vi "Encode_Decode Frame.vi"() -> ()   [LabVIEW 2020]
uses:
  Azdo/emea-aim-664-instrument-driver-1204/src/_controls/queue_data_full.ctl
  Azdo/emea-aim-664-instrument-driver-1204/src/_controls/queue_header_generic.ctl
  <vilib>/addons/_JKI Toolkits/Caraya/classes/Assert/Assert Equal Value_Variant.vi
  Azdo/emea-aim-664-instrument-driver-1204/src/AIM664LV.lvlib
  <vilib>/addons/_JKI Toolkits/Caraya/classes/Test/Test.lvclass
  <vilib>/addons/_JKI Toolkits/Caraya/classes/Assert/Assert.lvclass
panel:
  out "recv size":i32
  out "sent size":i32
  out "sent":u8[](array[numeric])
  out "recvd":u8[](array[numeric])
  in  "HeaderInfo":T1={"InterFrameGap"=0, "PacketGroupWaitTime"=10000, "PayloadBufferMode"=0, "PayloadGenerationMode"=0, "PreambleCount"=7, "Skew"=0, "NetSelect"=4, "FrameStartMode"=1, "PhysErrorInjection"=0, "SequenceNumberInit"=65535, "SequenceNumberOffset"=65535} {"NetSelect" items=["FDX_TX_FRAME_DLY_A"=0, "FDX_TX_FRAME_DLY_B"=1, "FDX_TX_FRAME_BOTH "=3, "FDX_TX_FRAME_ONLY_A"=4, "FDX_TX_FRAME_ONLY_B "=5]; "FrameStartMode" items=["FDX_TX_FRAME_START_IFG", "FDX_TX_FRAME_START_PGWT", "FDX_TX_FRAME_START_TRG"]; "PhysErrorInjection" items=["FDX_TX_FRAME_ERR_OFF"=0, "FDX_TX_FRAME_ERR_CRC"=1, "FDX_TX_FRAME_ERR_ALI"=2, "FDX_TX_FRAME_ERR_PRE"=4, "FDX_TX_FRAME_ERR_PHY"=8]; "SequenceNumberInit" items=["FDX_TX_FRAME_SEQ_INIT_AUTO"=65535]; "SequenceNumberOffset" items=["FDX_TX_FRAME_SEQ_OFFS_AUTO "=65535]; "PayloadGenerationMode" items=["FDX_TX_FRAME_PGM_USER"=0, "FDX_TX_FRAME_PGM_IP_PART"=1, "FDX_TX_FRAME_PGM_IP_FULL"=2, "FDX_TX_FRAME_PGM_IP_PART_TT"=10, "FDX_TX_FRAME_PGM_IP_FULL_TT"=20]; "PayloadBufferMode" items=["FDX_TX_FRAME_PBM_STD", "FDX_TX_FRAME_PBM_MAC", "FDX_TX_FRAME_PBM_UDP"]}
  in  "Frame payload size (bytes)":i32=100
  in  "UDPsrcPort":u16=1
  in  "Frame Configuration":T2={"domainID"=1, "sideID"=1, "locationID"=1, "interfaceID"=1, "partitionID"=1} {"interfaceID" format="%.0b"}
  in  "UDPdstPort":u16=1
  in  "VL Id":u16=60
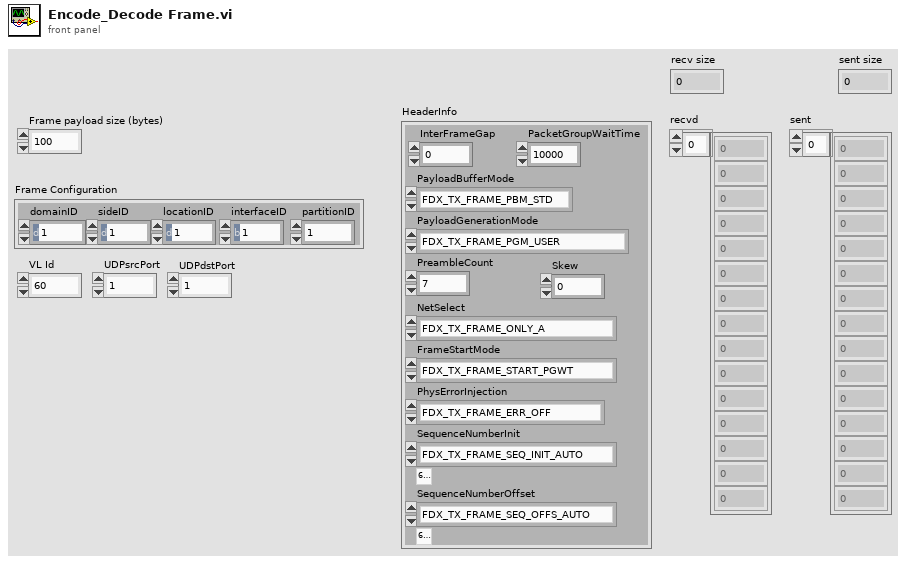
[diagram p1: front panel]
types:
  T1 = typedef "AIM664LV.lvlib/queue_header_generic.ctl" = cluster{"InterFrameGap":u32, "PacketGroupWaitTime":u32, "PayloadBufferMode":u8, "PayloadGenerationMode":u8, "PreambleCount":u8, "Skew":u32, "NetSelect":u8, "FrameStartMode":u8, "PhysErrorInjection":u32, "SequenceNumberInit":u16, "SequenceNumberOffset":u16}
  T2 = typedef "AIM664LV.lvlib/queue_data_full.ctl" = cluster{"domainID":u8, "sideID":u8, "locationID":u8, "interfaceID":u8, "partitionID":u8}
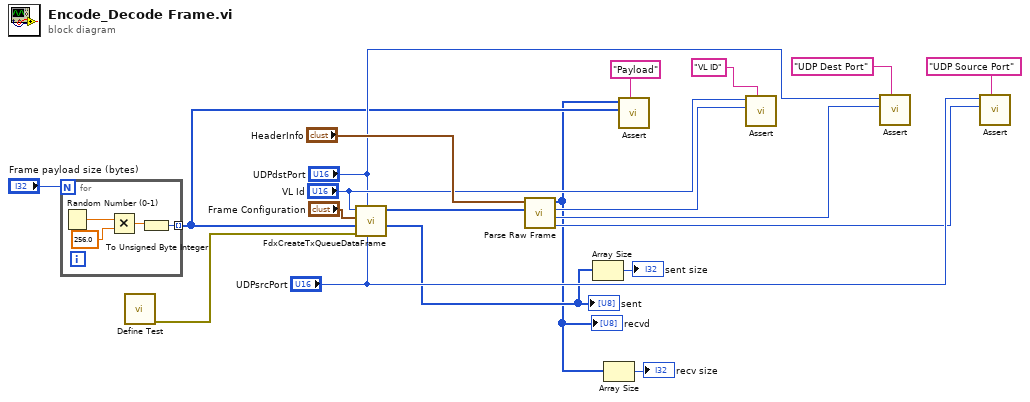
[diagram p0: block diagram]
diagram:
  n1 = for {
    N: "Frame payload size (bytes)" -> [_]
    tunnel: [w20] -> w4 mode=indexing
    n2 = Random Number (0-1)() -> (number: 0 to 1=w23:dbl)
    n3 = Multiply(x=w23, y=256.0) -> (x*y=w21:dbl)
    n4 = To Unsigned Byte Integer(number=w21) -> (unsigned 8bit integer=w20:u8)
  }
  "sent" <- w4
  n5 = call <vilib>:"Define Test.vi"() -> ("error out"=w5:errorcluster)  [unwired: 11 in]
  n6 = call "FdxCreateTxQueueDataFrame.vi"("UDPsrcPort"="UDPsrcPort", "UDPdstPort"="UDPdstPort", "error in"=w5, "Payload"=w4, "afdx configuration"="Frame Configuration", "VL Id"="VL Id") -> ("Frame"=w18:u8[])  [unwired: 3 in, 2 out]
  n7 = call "Parse Raw Frame.vi"("Data"=w18, "HeaderInfo"="HeaderInfo") -> ("UDPsrcPort"=w7:u16, "UDPdstPort"=w12:u16, "VL Id"=w15:u16, "Payload"=w1:u8[])  [unwired: 5 in, 1 out]
  "recvd" <- w1
  n8 = Array Size(array=w4) -> (size(s)=→"sent size":i32)
  n9 = Array Size(array=w1) -> (size(s)=→"recv size":i32)
  n10 = call-poly <vilib>:"Assert.vi"("Label"="Payload", "Y"=w4, "X"=w1) -> ()  [unwired: 8 in, 1 out]
  n11 = call-poly <vilib>:"Assert.vi"("Label"="VL ID", "Y"=w15, "X"="VL Id") -> ()  [unwired: 8 in, 1 out]
  n12 = call-poly <vilib>:"Assert.vi"("Label"="UDP Dest Port", "Y"=w12, "X"="UDPdstPort") -> ()  [unwired: 8 in, 1 out]
  n13 = call-poly <vilib>:"Assert.vi"("Label"="UDP Source Port", "Y"=w7, "X"="UDPsrcPort") -> ()  [unwired: 8 in, 1 out]
